vi "Offset_waveform_t0.vi"(8 "error in":errorcluster, 10 "t0":timestamp, 11 "Waveform array in":waveform(dbl)[](array[waveform])) -> (0 "error out":errorcluster, 3 "Waveform array out":waveform(dbl)[](array[waveform]))   [LabVIEW 2010]
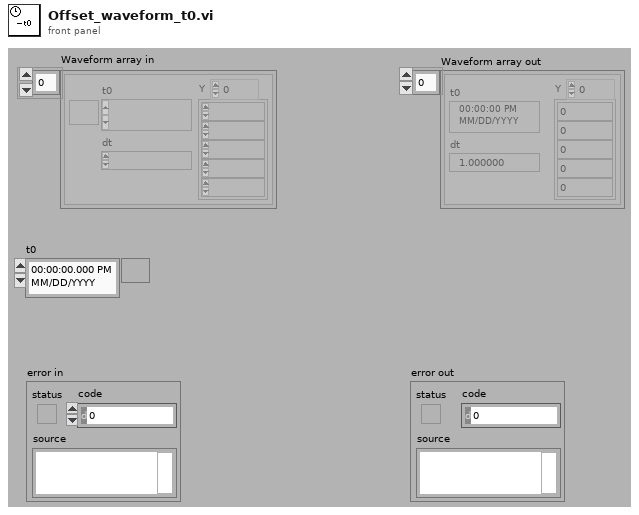
[diagram p1: front panel]
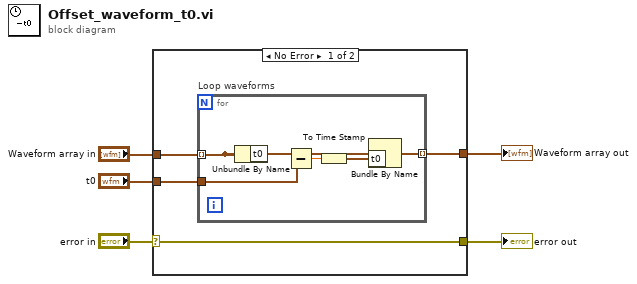
[diagram p0: block diagram]
diagram:
  n1 = case shown="No Error" "error in" {
    selector: "error in" -> [w9 w17]
    tunnel: [w9 w17] -> w4
    tunnel: "Waveform array in" -> [w8 w16]
    tunnel: "t0" -> [w7 _]
    tunnel: [w6 w16] -> w1
    frame No Error {
      n2 = for "Loop waveforms" {
        tunnel: w8 -> [w15] mode=indexing
        tunnel: w7 -> [w13]
        tunnel: [w10] -> w6 mode=indexing
        n3 = Unbundle By Name(w15) -> ("t0"=w14:timestamp)
        n4 = Subtract(x=w14, y=w13) -> (x-y=w12:dbl)
        n5 = To Time Stamp(1:w12) -> (0:w11:timestamp)
        n6 = Bundle By Name(cluster=w15, "t0"=w11) -> (w10:waveform(dbl))
      }
    }
    frame Error {
    }
  }
  "error out" <- w4
  "Waveform array out" <- w1
